vi "DSRead uint16.vi"(6 "wait for updated value (T)":bool, 8 "error in":errorcluster[](array[cluster]), 9 "ms timeout (10000)":i32, 11 "connection in":refnum<k13>[](array[refnum])) -> (0 "error out":errorcluster[](array[cluster]), 2 "data":u16[](array[numeric]), 3 "connection out":refnum<k13>[](array[refnum]))   [LabVIEW 2011]
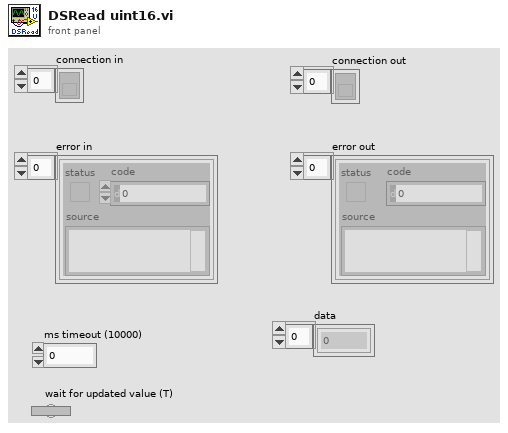
[diagram p1: front panel]
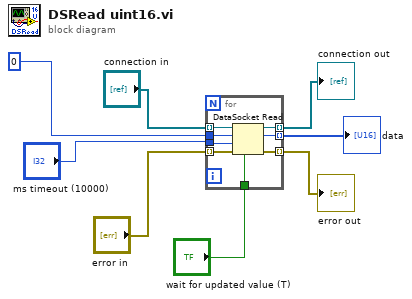
[diagram p0: block diagram]
diagram:
  n1 = for {
    tunnel: [w16] -> w5 mode=indexing
    tunnel: [w15] -> w6 mode=indexing
    tunnel: [w10] -> w2 mode=indexing
    tunnel: "connection in" -> [w14] mode=indexing
    tunnel: "error in" -> [w13] mode=indexing
    tunnel: "ms timeout (10000)" -> [w12]
    tunnel: "wait for updated value (T)" -> [w11]
    tunnel: u16 0 ("Numeric") -> [w9]
    n2 = DataSocket Read(6:w11, 8:w13, 9:w12, 10:w9, 11:w14) -> (0:w16:errorcluster, 2:w10:u16, 3:w15:refnum<k13>)  [unwired: 4 out]
  }
  "connection out" <- w6
  "error out" <- w5
  "data" <- w2
